vi "Autocross(1Lap).vi"() -> ()   [LabVIEW 2020]
uses:
  Control/AutocrossBestRecordIndicator.ctl
  Control/AutocrossCurrentRecordIndicator(1Lap).ctl
  Control/AutocrossState.ctl
  <vilib>/DAQmx/write.llb/DAQmx Write (Analog DBL 1Chan 1Samp).vi
  <vilib>/DAQmx/read.llb/DAQmx Read (Analog DBL 1Chan 1Samp).vi
  <vilib>/DAQmx/create/channels.llb/DAQmx Create Channel (AO-Voltage-Basic).vi
  <vilib>/DAQmx/create/channels.llb/DAQmx Create Channel (AI-Voltage-Basic).vi
  <vilib>/Utility/file.llb/Read Delimited Spreadsheet (string).vi
  <vilib>/DAQmx/miscellaneous.llb/DAQmx Fill In Error Info.vi
panel:
  out "Event Progress":string[][](table)
  in  "DeviceName":tag
  in  "NextButton":bool
  in  "Ready":bool
  in  "Retry":bool
  out "CurrentRecordIndicator":T1
  out "BestRecordIndicator":T2
  in  "Stop":bool
  # "2017 KSAE Formula Autocross Event"
  # "Time:"
  # "Entry:"
  # "#1"
  # "#2"
  # "#3"
  # "#4"
  # "Univ. :"
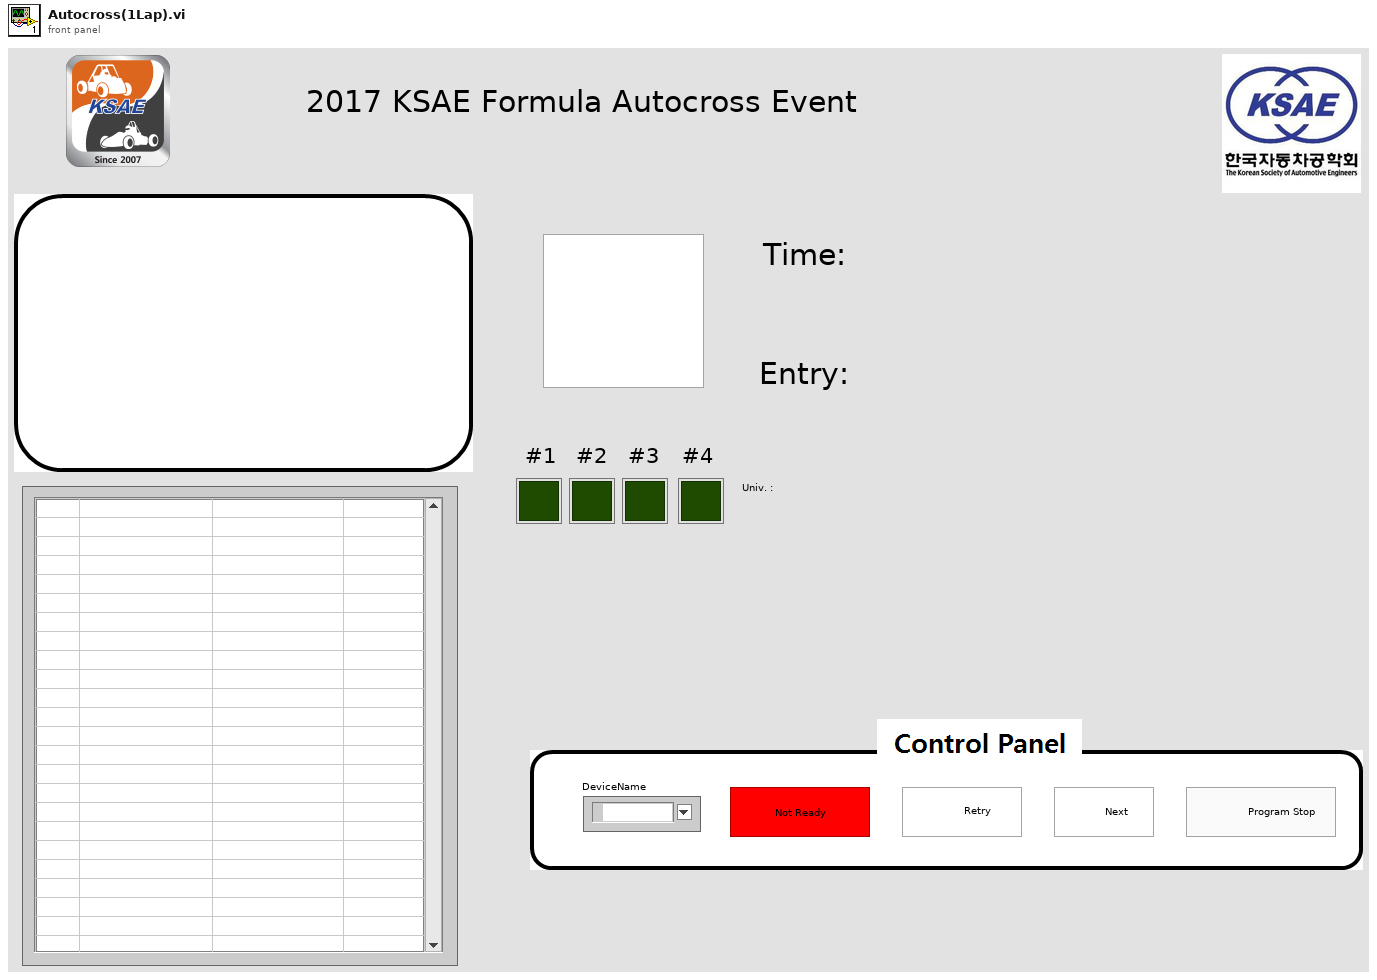
[diagram p1: front panel]
types:
  T1 = typedef "AutocrossCurrentRecordIndicator(1Lap).ctl" = cluster{"Time":string, "CurrentEntry":string, "CurrentUniversity":string, "Flag":picture, "CurrentState":string, "EventCount":cluster{"Attempt-1":bool, "Attempt-2":bool, "Attempt-3":bool, "Attempt-4":bool}}
  T2 = typedef "AutocrossBestRecordIndicator.ctl" = cluster{"BestSchool":string, "BestEntry":string, "BestTime":string}
  T3 = typedef "AutocrossState.ctl" = enum16{"Initial", "InputInfomation", "Ready", "1lap", "2lap", "FinshRunning", "LogRecord", "RenewBestRecord", "ProgramStop"}
  T4 = cluster{"CurrentRecordIndicator":T1, "BestRecordIndicator":T2, "FlageData":cluster{"GreenFlag":picture, "BlueFlag":picture, "RedFlag":picture}, "1LapRefTime":i64, "1LapTime":i64, "State":T3, "EventProgressData":string[][], "EventCount":i32}
  T5 = cluster{"CurrentEntry":string, "CurrentUniversity":string, "CurrentTeam":string}
  T6 = cluster{"Attempt-1":bool, "Attempt-2":bool, "Attempt-3":bool, "Attempt-4":bool}
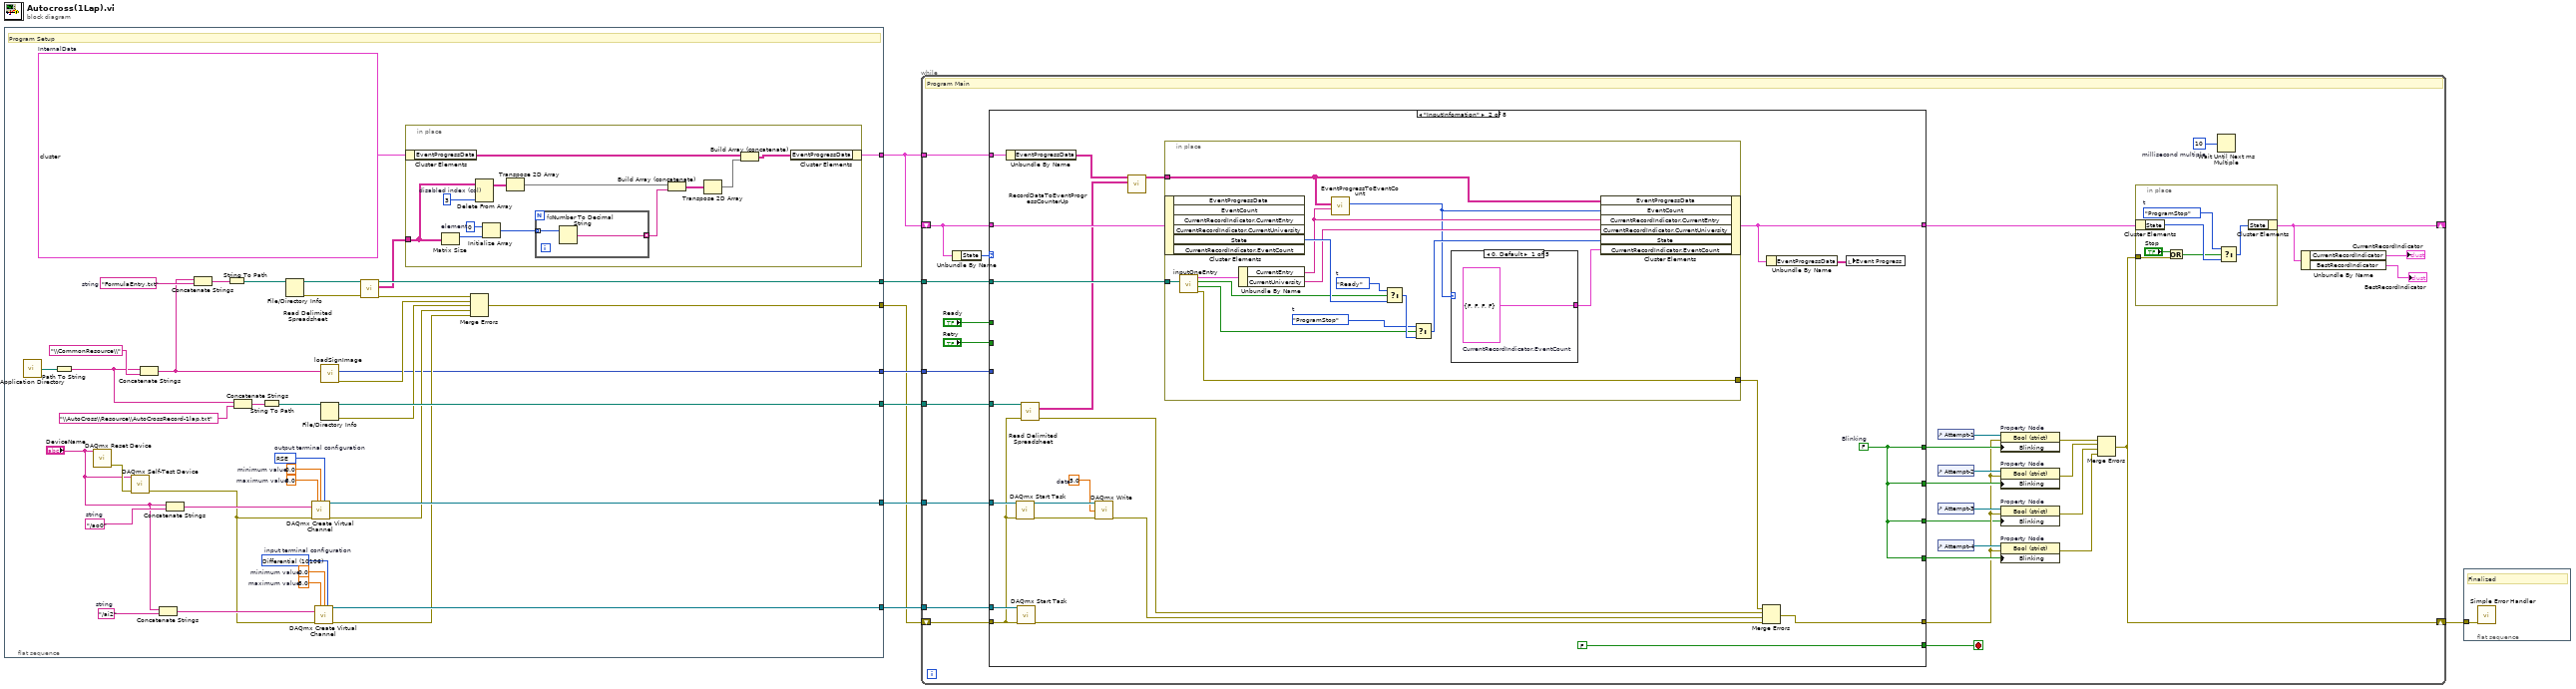
[diagram p0: block diagram]
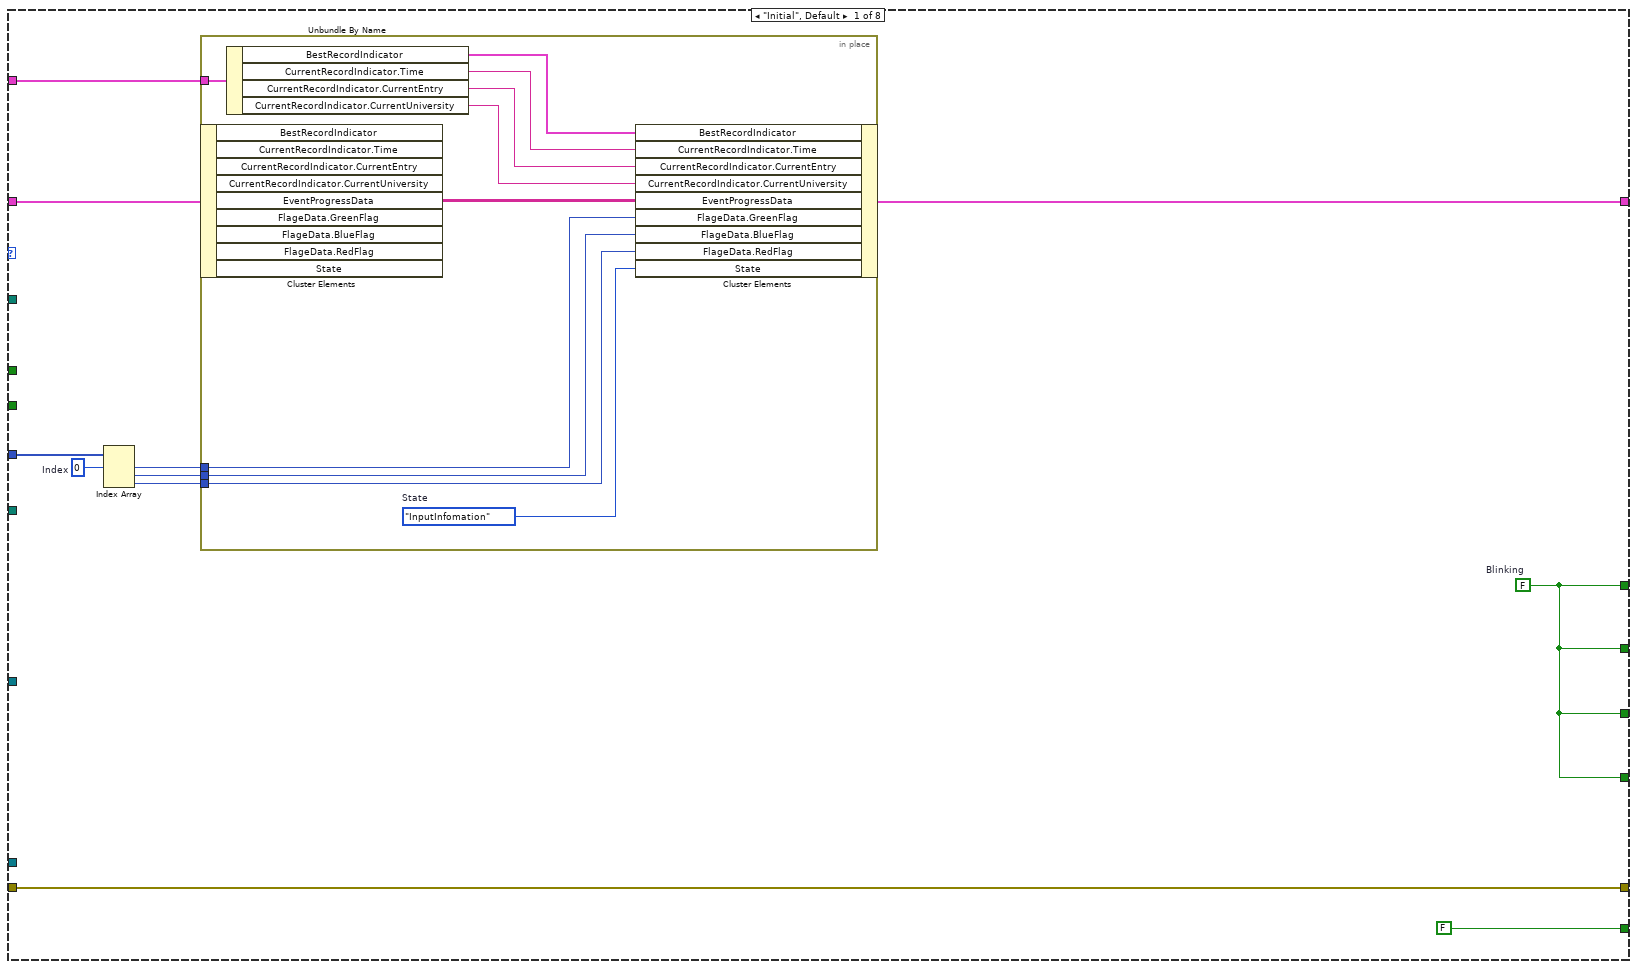
[diagram p2: hidden frame]
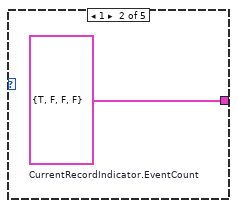
[diagram p3: hidden frame]
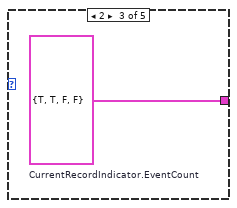
[diagram p4: hidden frame]
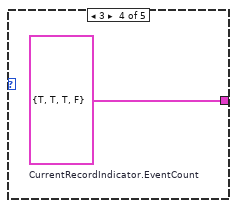
[diagram p5: hidden frame]
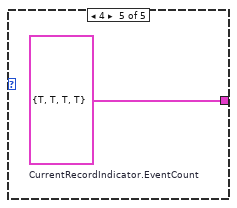
[diagram p6: hidden frame]
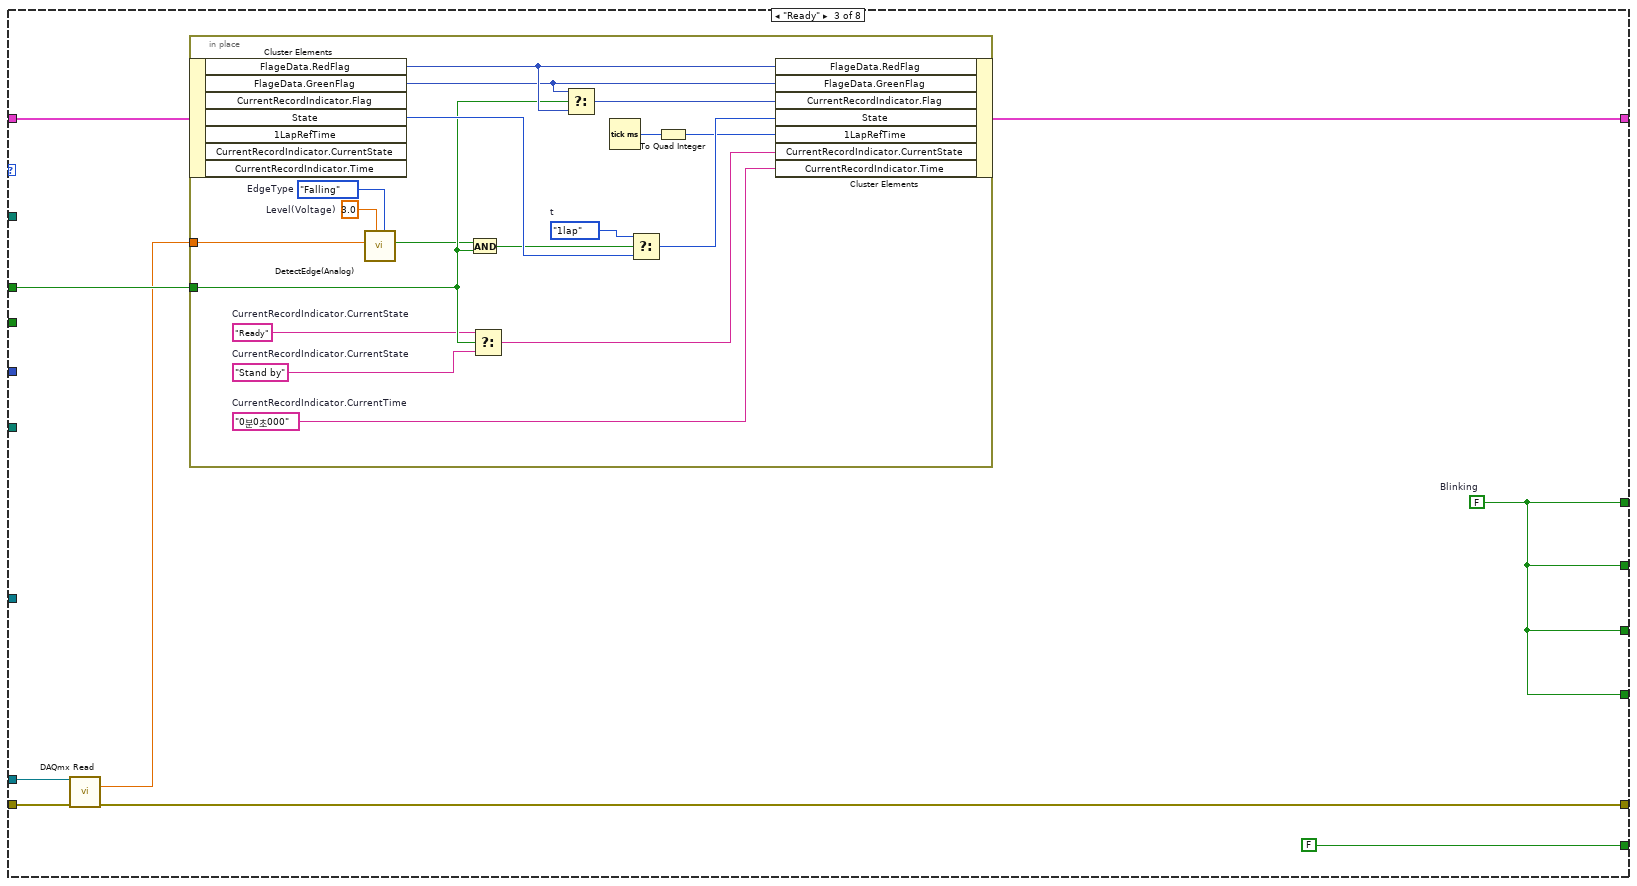
[diagram p7: hidden frame]
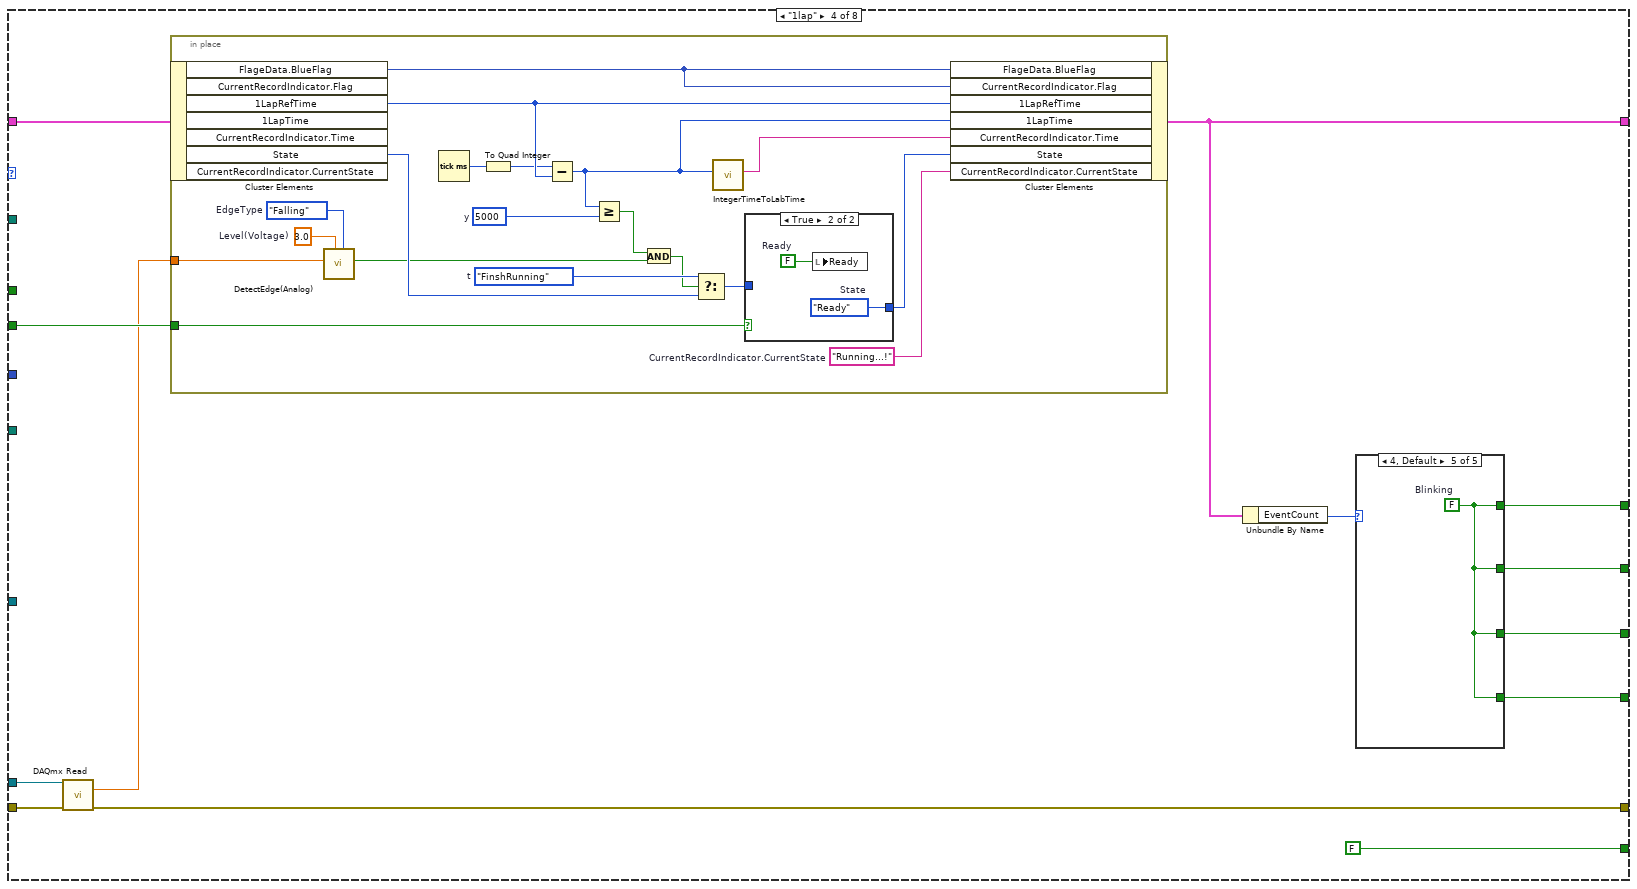
[diagram p8: hidden frame]
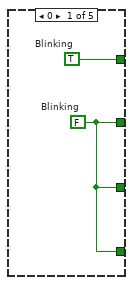
[diagram p9: hidden frame]
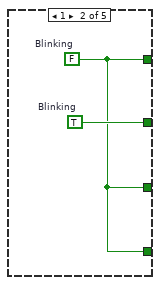
[diagram p10: hidden frame]
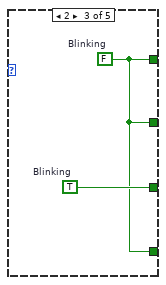
[diagram p11: hidden frame]
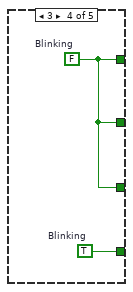
[diagram p12: hidden frame]
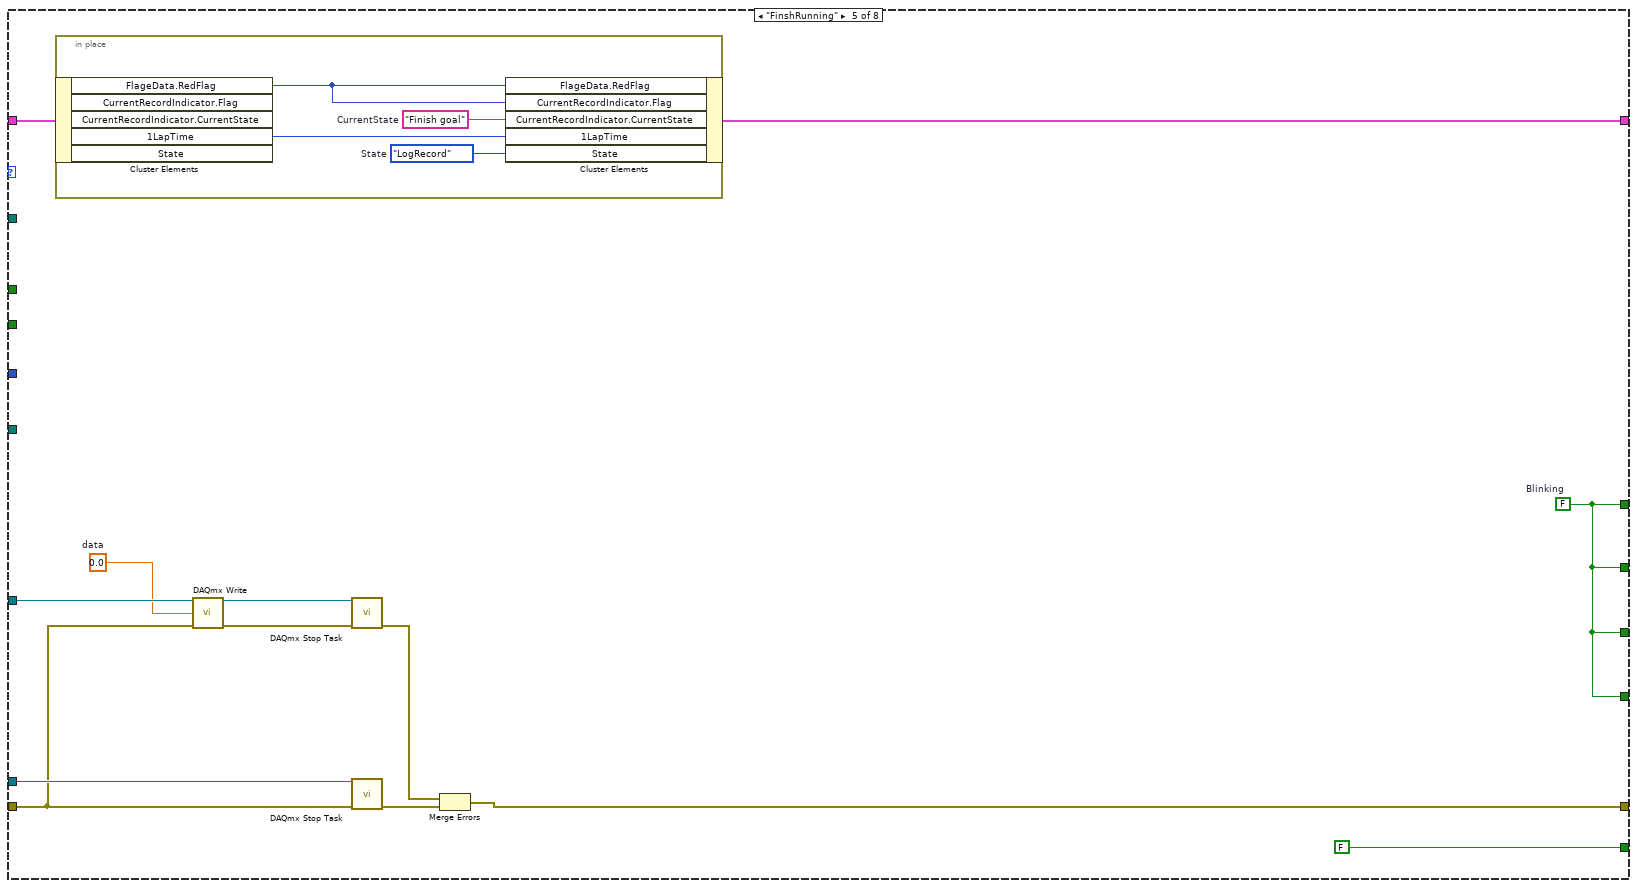
[diagram p14: hidden frame]
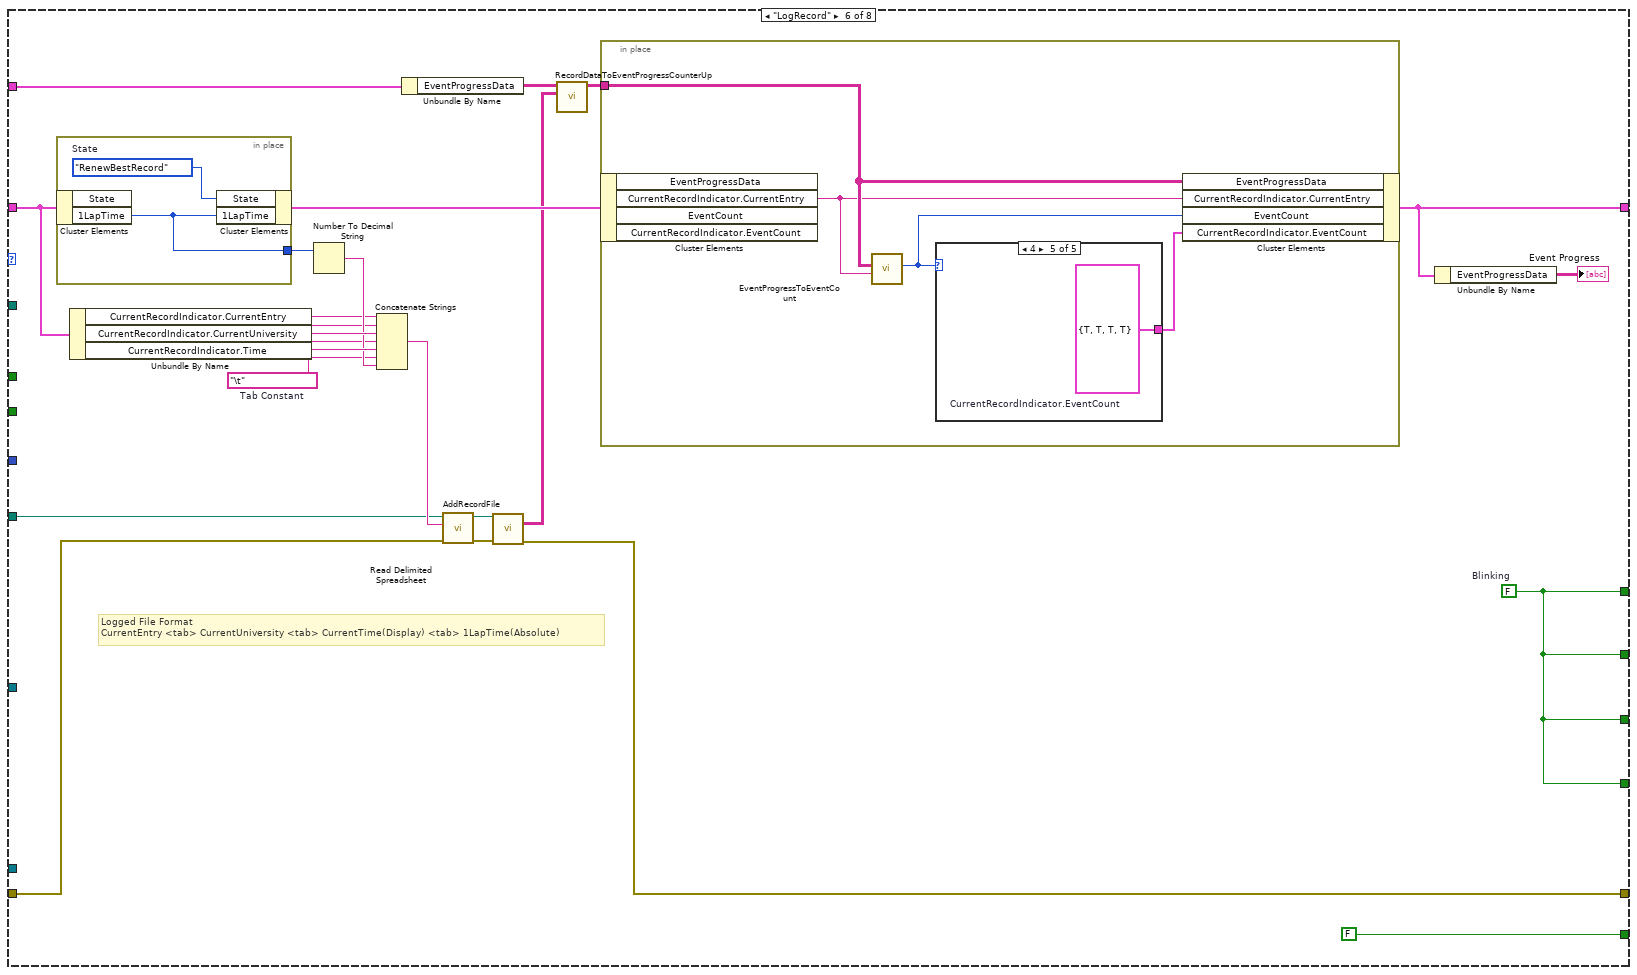
[diagram p15: hidden frame]
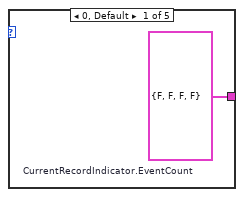
[diagram p16: hidden frame]
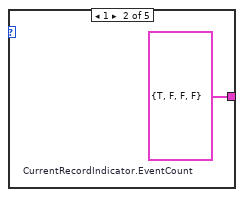
[diagram p17: hidden frame]
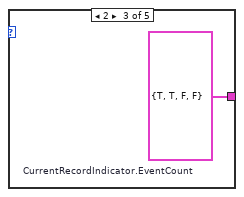
[diagram p18: hidden frame]
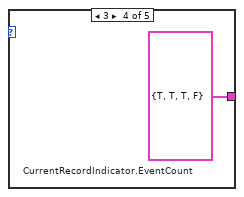
[diagram p19: hidden frame]
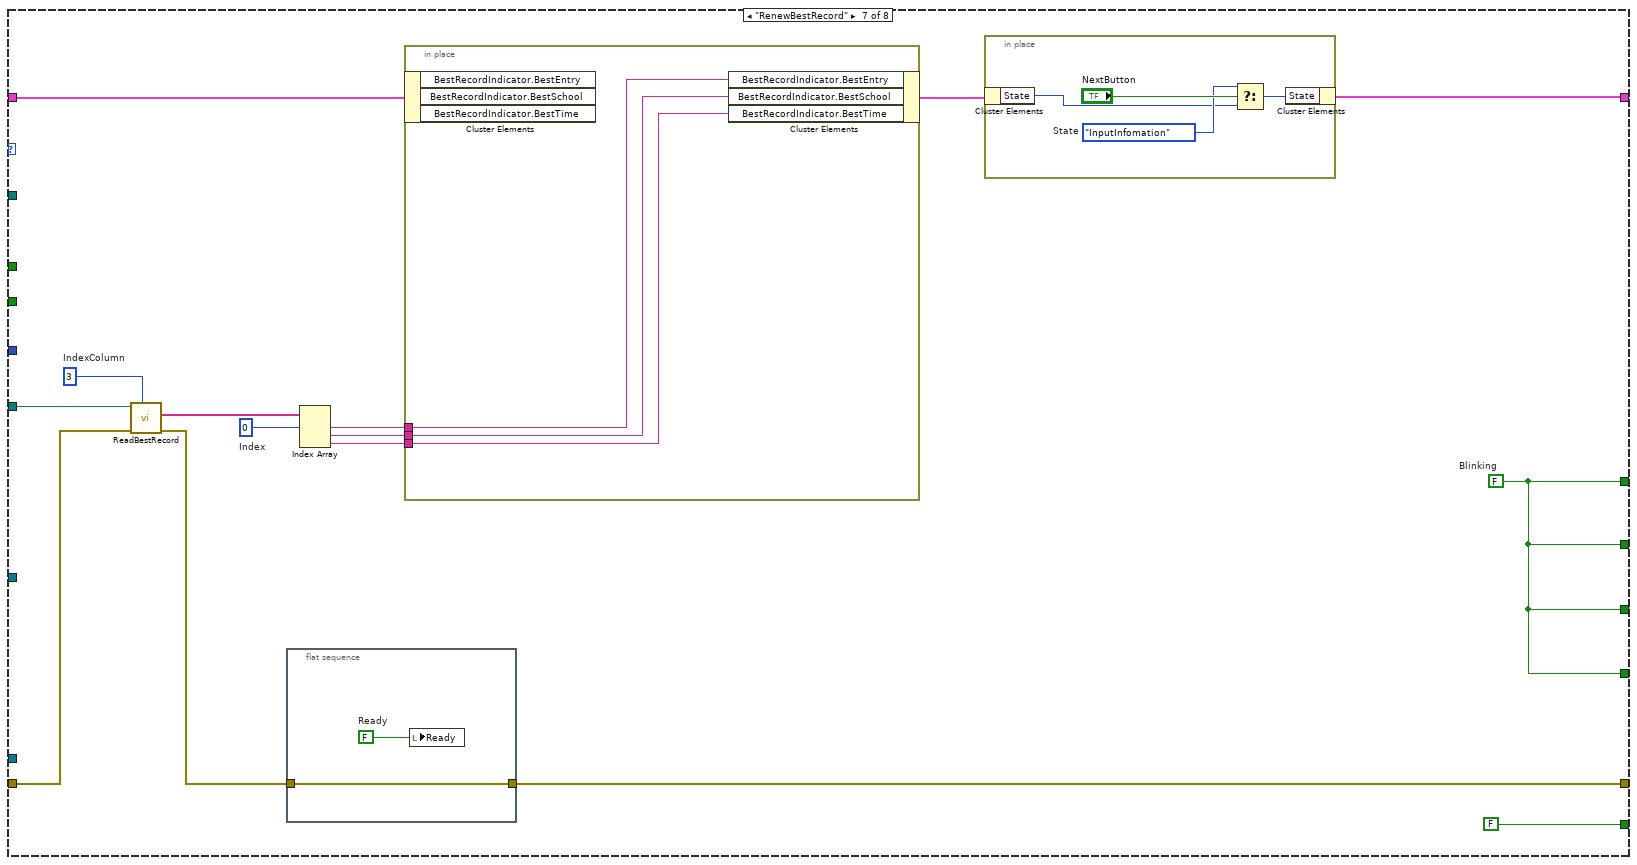
[diagram p20: hidden frame]
diagram:
  n1 = flat-sequence {
    tunnel: [w13] -> w7
    tunnel: [w46] -> w6
    tunnel: [w43] -> w5
    tunnel: [w23] -> w4
    tunnel: [w9] -> w3
    tunnel: [w24] -> w2
    tunnel: [w16] -> w1
    frame #0 {
      w15 = T4 {"CurrentRecordIndicator"={"Time"="", "CurrentEntry"="", "CurrentUniversity"="", "Flag"=bytes[0], "CurrentState"="", "EventCount"={"Attempt-1"=FALSE, "Attempt-2"=FALSE, "Attempt-3"=FALSE, "Attempt-4"=FALSE}}, "BestRecordIndicator"={"BestSchool"="", "BestEntry"="", "BestTime"=""}, "FlageData"={"GreenFlag"=bytes[0], "BlueFlag"=bytes[0], "RedFlag"=bytes[0]}, "1LapRefTime"=0, "1LapTime"=0, "State"=enum."Initial", "EventProgressData"=[["Entry ", "University", "Team", "Event Count"]], "EventCount"=0}  # InternalData
      w31 = "/ai2"  # string
      w32 = "/ao0"  # string
      w33 = "FormulaEntry.txt"  # string
      w40 = 10083 items=["Default"=-1, "RSE"=10083, "Differential"=10106, "Pseudodifferential"=12529]  # output terminal configuration
      w41 = 0.0  # minimum value
      w42 = 5.0  # maximum value
      w45 = 5.0  # maximum value
      w44 = 0.0  # minimum value
      w47 = 10106 items=["default"=-1, "RSE"=10083, "NRSE"=10078, "Differential"=10106, "Pseudodifferential"=12529]  # input terminal configuration
      # "Program Setup"
      n2 = call <vilib>:"Application Directory.vi"() -> ("Application Directory"=w39:path)
      n3 = Path To String(path=w39) -> (string=w35:string)
      n4 = call <vilib>:"DAQmx Reset Device.vi"("device in"="DeviceName") -> ("error out"=w12:errorcluster)  [unwired: 14 in]
      n5 = call <vilib>:"DAQmx Self-Test Device.vi"("device in"="DeviceName", "error in"=w12) -> ("error out"=w11:errorcluster)  [unwired: 13 in]
      n6 = Concatenate Strings "Concatenate Strings"(w35, "\\CommonResource\\") -> (w26:string)
      n7 = Concatenate Strings "Concatenate Strings"("DeviceName", w31) -> (w29:string)
      n8 = Concatenate Strings "Concatenate Strings"("DeviceName", w32) -> (w30:string)
      n9 = Concatenate Strings "Concatenate Strings"(w26, w33) -> (w34:string)
      n10 = String To Path(string=w34) -> (path=w28:path)
      n11 = Concatenate Strings "Concatenate Strings"(w35, "\\AutoCross\\Resource\\AutoCrossRecord-1lap.txt") -> (w37:string)
      n12 = String To Path(string=w37) -> (path=w25:path)
      n13 = File/Directory Info(path=w28) -> (path out=w27:path, error out=w22:errorcluster)  [unwired: 1 in, 5 out]
      n14 = call-poly <vilib>:"DAQmx Create Virtual Channel.vi"("maximum value"=w42, "minimum value"=w41, "output terminal configuration"=w40, "physical channels"=w30, "error in"=w11) -> ("task out"=w43:refnum<k21>, "error out"=w18:errorcluster)  [unwired: 9 in]
      n15 = call-poly <vilib>:"DAQmx Create Virtual Channel.vi"("maximum value"=w45, "minimum value"=w44, "input terminal configuration"=w47, "physical channels"=w29, "error in"=w11) -> ("task out"=w46:refnum<k21>, "error out"=w17:errorcluster)  [unwired: 9 in]
      n16 = File/Directory Info(path=w25) -> (path out=w23:path, error out=w19:errorcluster)  [unwired: 1 in, 5 out]
      n17 = call "loadSignImage.vi"("String"=w26) -> ("outputError"=w20:errorcluster, "SignImageOutput"=w9:picture[])  [unwired: 9 in]
      n18 = call-poly <vilib>:"Read Delimited Spreadsheet.vi"("file path (dialog if empty)"=w27, "error in (no error)"=w22) -> ("new file path (Not A Path if cancelled)"=w24:path, "all rows"=w14:string[][], "error out"=w21:errorcluster)  [unwired: 8 in, 3 out]
      n19 = in-place {
        in-place-border: w14 -> [w56]
        w55 = 3  # disabled index (col)
        w58 = 0  # element
        n20 = in-place-cluster #1(w15) -> ("EventProgressData"=w49:string[][])
        n21 = Matrix Size(0:w56) -> (1:w59:i32)  [unwired: 1 out]
        n22 = Delete From Array "Delete From Array"(array=w56, index (col)=w55) -> (array with subset deleted=w54:string[][])  [unwired: 2 in, 1 out]
        n23 = Initialize Array "Initialize Array"(w58, w59) -> (w57:i32[])
        n24 = Transpose 2D Array(2D array=w54) -> (transposed array=w53:string[][])
        n25 = for {
          tunnel: w57 -> [w61] mode=indexing
          tunnel: [w60] -> w52 mode=indexing
          n26 = Number To Decimal String(number=w61) -> (decimal integer string=w60:string)  [unwired: 1 in]
        }
        n27 = Build Array (concatenate) "Build Array"(w53, w52) -> (w51:string[][])
        n28 = Transpose 2D Array(2D array=w51) -> (transposed array=w50:string[][])
        n29 = Build Array (concatenate) "Build Array"(w49, w50) -> (w48:string[][])
        n30 = in-place-cluster #1("EventProgressData"=w48) -> (w13:T4)
      }
      n31 = Merge Errors "Merge Errors"(w21, w20, w19, w18, w17) -> (w16:errorcluster)
    }
  }
  n32 = while {
    tunnel: w6 -> [w92]
    shift-right: [w85] -> _
    shift-left: w7 -> [w89]
    shift-right: [w63] -> w8
    shift-left: w1 -> [w91]
    tunnel: w7 -> [w83]
    tunnel: w5 -> [w80]
    tunnel: w4 -> [w79]
    tunnel: w3 -> [w77]
    tunnel: w2 -> [w76]
    stop <- w84 stop-if-true
    w78 = u32 10  # millisecond multiple
    # "Program Main"
    n33 = Unbundle By Name(w89) -> ("State"=w90:T3)
    n34 = case shown="\"InputInfomation\"" w90 {
      tunnel: w92 -> [_ w134 w164 w195 w239 _ _ w308]
      tunnel: w91 -> [w94 w115 w163 w194 w228 w255 w289 w302]
      tunnel: w89 -> [w103 w135 w162 w193 w238 w264 w291 w310]
      tunnel: [w102 w117 w161 w188 w237 w245 w281 w309] -> w86
      tunnel: [FALSE FALSE FALSE FALSE FALSE FALSE FALSE TRUE] -> w84
      tunnel: [w94 w132 w160 w192 w232 w248 w279 w304] -> w68
      tunnel: w83 -> [w96 w121 _ _ _ w252 _ _]
      tunnel: "Ready" -> [_ _ w159 _ _ _ _ _]
      tunnel: "Retry" -> [_ _ _ w191 _ _ _ _]
      tunnel: w80 -> [_ w131 _ _ w235 _ _ w305]
      tunnel: w79 -> [_ w123 _ _ _ w258 w278 _]
      tunnel: w77 -> [w95 _ _ _ _ _ _ _]
      tunnel: w76 -> [_ w124 _ _ _ _ _ _]
      tunnel: [w93 w114 w156 w186 w227 w244 w277 w301] -> w71
      tunnel: [w93 w114 w156 w185 w227 w244 w277 w301] -> w70
      tunnel: [w93 w114 w156 w183 w227 w244 w277 w301] -> w69
      tunnel: [w93 w114 w156 w184 w227 w244 w277 w301] -> w62
      frame "Initial", Default {
        w93 = FALSE  # Blinking
        w97 = 0  # Index
        n35 = Index Array "Index Array"(array=w95, index #1=w97) -> (element #1=w100:picture, element #2=w99:picture, element #3=w98:picture)  [unwired: 2 in]
        n36 = in-place {
          in-place-border: w100 -> [w113]
          in-place-border: w99 -> [w112]
          in-place-border: w98 -> [w111]
          in-place-border: w96 -> [w109]
          w110 = AutocrossState."InputInfomation"  # State
          n37 = in-place-cluster #2(w103) -> ("EventProgressData"=w104:string[][])  [unwired: 8 out]
          n38 = Unbundle By Name(w109) -> ("BestRecordIndicator"=w108:T2, "CurrentRecordIndicator.Time"=w107:string, "CurrentRecordIndicator.CurrentEntry"=w105:string, "CurrentRecordIndicator.CurrentUniversity"=w106:string)
          n39 = in-place-cluster #2("BestRecordIndicator"=w108, "CurrentRecordIndicator.Time"=w107, "CurrentRecordIndicator.CurrentEntry"=w105, "CurrentRecordIndicator.CurrentUniversity"=w106, "EventProgressData"=w104, "FlageData.GreenFlag"=w113, "FlageData.BlueFlag"=w112, "FlageData.RedFlag"=w111, "State"=w110) -> (w102:T4)
        }
      }
      frame "InputInfomation" {
        w114 = FALSE  # Blinking
        w126 = 5.0  # data
        n40 = Unbundle By Name(w121) -> ("EventProgressData"=w120:string[][])
        n41 = call <vilib>:"DAQmx Start Task.vi"("task/channels in"=w131, "error in"=w115) -> ("task out"=w129:refnum<k21>, "error out"=w128:errorcluster)  [unwired: 12 in]
        n42 = call <vilib>:"DAQmx Start Task.vi"("task/channels in"=w134, "error in"=w115) -> ("error out"=w133:errorcluster)  [unwired: 12 in, 1 out]
        n43 = call-poly <vilib>:"Read Delimited Spreadsheet.vi"("file path (dialog if empty)"=w123, "error in (no error)"=w115) -> ("all rows"=w119:string[][], "error out"=w122:errorcluster)  [unwired: 8 in, 4 out]
        n44 = call-poly <vilib>:"DAQmx Write.vi"("task/channels in"=w129, "data"=w126, "error in"=w128) -> ("error out"=w127:errorcluster)  [unwired: 10 in, 2 out]
        n45 = call "RecordDataToEventProgressCounterUp.vi"("RecordData"=w119, "EventProgressDataInput"=w120) -> ("EventProgressDataOutput"=w118:string[][])  [unwired: 9 in]
        n46 = in-place {
          in-place-border: [w145] -> w130
          in-place-border: w124 -> [w138]
          in-place-border: w118 -> [w143]
          w147 = AutocrossState."ProgramStop"  # t
          w149 = AutocrossState."Ready"  # t
          n47 = in-place-cluster #3(w135) -> ("State"=w150:T3)  [unwired: 5 out]
          n48 = call "inputOneEntry.vi"("file path (dialog if empty)"=w138) -> ("outputError"=w145:errorcluster, "StopButtonOutput"=w136:bool, "OKButtonOutput"=w137:bool, "CurrentData"=w139:T5)  [unwired: 7 in]
          n49 = Unbundle By Name(w139) -> ("CurrentEntry"=w142:string, "CurrentUniversity"=w144:string)
          n50 = call "EventProgressToEventCount.vi"("CurrentEntry"=w142, "EventProgressDataInput"=w143) -> ("EventCount"=w141:i32)  [unwired: 9 in]
          n51 = Select(t=w149, s=w137, f=w150) -> (s? t:f=w148:T3)
          n52 = Select(t=w147, s=w136, f=w148) -> (s? t:f=w146:T3)
          n53 = case shown="0, Default" w141 {
            tunnel: [w151 w152 w153 w154 w155] -> w140
            frame 0, Default {
              w151 = T6 {"Attempt-1"=FALSE, "Attempt-2"=FALSE, "Attempt-3"=FALSE, "Attempt-4"=FALSE}  # CurrentRecordIndicator.EventCount
            }
            frame 1 {
              w152 = T6 {"Attempt-1"=TRUE, "Attempt-2"=FALSE, "Attempt-3"=FALSE, "Attempt-4"=FALSE}  # CurrentRecordIndicator.EventCount
            }
            frame 2 {
              w153 = T6 {"Attempt-1"=TRUE, "Attempt-2"=TRUE, "Attempt-3"=FALSE, "Attempt-4"=FALSE}  # CurrentRecordIndicator.EventCount
            }
            frame 3 {
              w154 = T6 {"Attempt-1"=TRUE, "Attempt-2"=TRUE, "Attempt-3"=TRUE, "Attempt-4"=FALSE}  # CurrentRecordIndicator.EventCount
            }
            frame 4 {
              w155 = T6 {"Attempt-1"=TRUE, "Attempt-2"=TRUE, "Attempt-3"=TRUE, "Attempt-4"=TRUE}  # CurrentRecordIndicator.EventCount
            }
          }
          n54 = in-place-cluster #3("EventProgressData"=w143, "EventCount"=w141, "CurrentRecordIndicator.CurrentEntry"=w142, "CurrentRecordIndicator.CurrentUniversity"=w144, "State"=w146, "CurrentRecordIndicator.EventCount"=w140) -> (w117:T4)
        }
        n55 = Merge Errors "Merge Errors"(w130, w122, w127, w133) -> (w132:errorcluster)
        n56 = Unbundle By Name(w117) -> ("EventProgressData"=w116:string[][])
        n57 = local write "Event Progress"(w116) -> ()
      }
      frame "Ready" {
        w156 = FALSE  # Blinking
        n58 = call-poly <vilib>:"DAQmx Read.vi"("task/channels in"=w164, "error in"=w163) -> ("data"=w158:dbl, "error out"=w160:errorcluster)  [unwired: 11 in, 1 out]
        n59 = in-place {
          in-place-border: w158 -> [w179]
          in-place-border: w159 -> [w173]
          w165 = enum16{"Rising", "Falling"}."Falling"  # EdgeType
          w170 = "Stand by"  # CurrentRecordIndicator.CurrentState
          w174 = 3.0  # Level(Voltage)
          w167 = "0분0초000"  # CurrentRecordIndicator.CurrentTime
          w171 = "Ready"  # CurrentRecordIndicator.CurrentState
          w180 = AutocrossState."1lap"  # t
          n60 = in-place-cluster #4(w162) -> ("FlageData.RedFlag"=w176:picture, "FlageData.GreenFlag"=w175:picture, "State"=w182:T3)  [unwired: 4 out]
          n61 = call "DetectEdge(Analog).vi"("EdgeType"=w165, "Level(Voltage)"=w174, "Voltage"=w179) -> ("DetectedEdge"=w166:bool)  [unwired: 8 in]
          n62 = And(x=w166, y=w173) -> (x .and. y?=w178:bool)
          n63 = Select(t=w171, s=w173, f=w170) -> (s? t:f=w172:string)
          n64 = Select(t=w175, s=w173, f=w176) -> (s? t:f=w177:picture)
          n65 = Tick Count (ms)() -> (millisecond timer value=w169:u32)
          n66 = Select(t=w180, s=w178, f=w182) -> (s? t:f=w181:T3)
          n67 = To Quad Integer(1:w169) -> (0:w168:i64)
          n68 = in-place-cluster #4("FlageData.RedFlag"=w176, "FlageData.GreenFlag"=w175, "CurrentRecordIndicator.Flag"=w177, "State"=w181, "1LapRefTime"=w168, "CurrentRecordIndicator.CurrentState"=w172, "CurrentRecordIndicator.Time"=w167) -> (w161:T4)
        }
      }
      frame "1lap" {
        n69 = call-poly <vilib>:"DAQmx Read.vi"("task/channels in"=w195, "error in"=w194) -> ("data"=w190:dbl, "error out"=w192:errorcluster)  [unwired: 11 in, 1 out]
        n70 = in-place {
          in-place-border: w191 -> [w209]
          in-place-border: w190 -> [w219]
          w205 = enum16{"Rising", "Falling"}."Falling"  # EdgeType
          w210 = i64 5000  # y
          w218 = 3.0  # Level(Voltage)
          w221 = "Running...!"  # CurrentRecordIndicator.CurrentState
          w223 = AutocrossState."FinshRunning"  # t
          n71 = in-place-cluster #5(w193) -> ("FlageData.BlueFlag"=w222:picture, "1LapRefTime"=w216:i64, "State"=w213:T3)  [unwired: 4 out]
          n72 = call "DetectEdge(Analog).vi"("EdgeType"=w205, "Level(Voltage)"=w218, "Voltage"=w219) -> ("DetectedEdge"=w207:bool)  [unwired: 8 in]
          n73 = Tick Count (ms)() -> (millisecond timer value=w217:u32)
          n74 = To Quad Integer(1:w217) -> (0:w215:i64)
          n75 = Subtract(x=w215, y=w216) -> (x-y=w211:i64)
          n76 = Greater Or Equal?(x=w211, y=w210) -> (x >= y?=w208:bool)
          n77 = And(x=w208, y=w207) -> (x .and. y?=w206:bool)
          n78 = Select(t=w223, s=w206, f=w213) -> (s? t:f=w220:T3)
          n79 = call "IntegerTimeToLabTime.vi"("inputTime(msec)"=w211) -> ("outputTime(mm-ss-sss)"=w214:string)  [unwired: 10 in]
          n80 = case shown="True" w209 {
            tunnel: w220 -> [w224 _]
            tunnel: [w224 w225] -> w212
            frame False {
            }
            frame True {
              w225 = AutocrossState."Ready"  # State
              w226 = FALSE  # Ready
              n81 = local write "Ready"(w226) -> ()
            }
          }
          n82 = in-place-cluster #5("FlageData.BlueFlag"=w222, "CurrentRecordIndicator.Flag"=w222, "1LapRefTime"=w216, "1LapTime"=w211, "CurrentRecordIndicator.Time"=w214, "State"=w212, "CurrentRecordIndicator.CurrentState"=w221) -> (w188:T4)
        }
        n83 = Unbundle By Name(w188) -> ("EventCount"=w187:i32)
        n84 = case shown="4, Default" w187 {
          tunnel: [w197 w198 w200 w202 w204] -> w186
          tunnel: [w196 w199 w200 w202 w204] -> w185
          tunnel: [w196 w198 w201 w202 w204] -> w184
          tunnel: [w196 w198 w200 w203 w204] -> w183
          frame 0 {
            w196 = FALSE  # Blinking
            w197 = TRUE  # Blinking
          }
          frame 1 {
            w199 = TRUE  # Blinking
            w198 = FALSE  # Blinking
          }
          frame 2 {
            w201 = TRUE  # Blinking
            w200 = FALSE  # Blinking
          }
          frame 3 {
            w203 = TRUE  # Blinking
            w202 = FALSE  # Blinking
          }
          frame 4, Default {
            w204 = FALSE  # Blinking
          }
        }
      }
      frame "FinshRunning" {
        w227 = FALSE  # Blinking
        w230 = 0.0  # data
        n85 = in-place {
          w241 = AutocrossState."LogRecord"  # State
          w242 = "Finish goal"  # CurrentState
          n86 = in-place-cluster #6(w238) -> ("FlageData.RedFlag"=w243:picture, "1LapTime"=w240:i64)  [unwired: 3 out]
          n87 = in-place-cluster #6("FlageData.RedFlag"=w243, "CurrentRecordIndicator.Flag"=w243, "CurrentRecordIndicator.CurrentState"=w242, "1LapTime"=w240, "State"=w241) -> (w237:T4)
        }
        n88 = call-poly <vilib>:"DAQmx Write.vi"("task/channels in"=w235, "data"=w230, "error in"=w228) -> ("task out"=w234:refnum<k21>, "error out"=w233:errorcluster)  [unwired: 10 in, 1 out]
        n89 = call <vilib>:"DAQmx Stop Task.vi"("task/channels in"=w234, "error in"=w233) -> ("error out"=w231:errorcluster)  [unwired: 12 in, 1 out]
        n90 = call <vilib>:"DAQmx Stop Task.vi"("task/channels in"=w239, "error in"=w228) -> ("error out"=w236:errorcluster)  [unwired: 12 in, 1 out]
        n91 = Merge Errors "Merge Errors"(w231, w236) -> (w232:errorcluster)
      }
      frame "LogRecord" {
        w244 = FALSE  # Blinking
        w259 = "\t"  # Tab Constant
        # "Logged File Format\nCurrentEntry <tab> CurrentUniversity <tab> CurrentTime(Display) <tab> 1LapTime(Absolute)"
        n92 = in-place {
          in-place-border: [w275] -> w254
          w276 = AutocrossState."RenewBestRecord"  # State
          n93 = in-place-cluster #7(w264) -> ("1LapTime"=w275:i64)  [unwired: 1 out]
          n94 = in-place-cluster #7("State"=w276, "1LapTime"=w275) -> (w253:T4)
        }
        n95 = Unbundle By Name(w264) -> ("CurrentRecordIndicator.CurrentEntry"=w257:string, "CurrentRecordIndicator.CurrentUniversity"=w263:string, "CurrentRecordIndicator.Time"=w262:string)
        n96 = Number To Decimal String(number=w254) -> (decimal integer string=w260:string)  [unwired: 1 in]
        n97 = Concatenate Strings "Concatenate Strings"(w257, w259, w263, w259, w262, w259, w260) -> (w261:string)
        n98 = Unbundle By Name(w252) -> ("EventProgressData"=w251:string[][])
        n99 = call "AddRecordFile.vi"("에러 입력"=w255, "LabTime"=w261, "파일 경로(대화 상자 사용)"=w258) -> ("에러 출력"=w249:errorcluster, "경로"=w250:path)  [unwired: 7 in]
        n100 = call-poly <vilib>:"Read Delimited Spreadsheet.vi"("file path (dialog if empty)"=w250, "error in (no error)"=w249) -> ("all rows"=w247:string[][], "error out"=w248:errorcluster)  [unwired: 8 in, 4 out]
        n101 = call "RecordDataToEventProgressCounterUp.vi"("RecordData"=w247, "EventProgressDataInput"=w251) -> ("EventProgressDataOutput"=w246:string[][])  [unwired: 9 in]
        n102 = in-place {
          in-place-border: w246 -> [w269]
          n103 = in-place-cluster #8(w253) -> ("CurrentRecordIndicator.CurrentEntry"=w268:string)  [unwired: 3 out]
          n104 = call "EventProgressToEventCount.vi"("CurrentEntry"=w268, "EventProgressDataInput"=w269) -> ("EventCount"=w267:i32)  [unwired: 9 in]
          n105 = case shown="4" w267 {
            tunnel: [w270 w271 w272 w273 w274] -> w266
            frame 0, Default {
              w270 = T6 {"Attempt-1"=FALSE, "Attempt-2"=FALSE, "Attempt-3"=FALSE, "Attempt-4"=FALSE}  # CurrentRecordIndicator.EventCount
            }
            frame 1 {
              w271 = T6 {"Attempt-1"=TRUE, "Attempt-2"=FALSE, "Attempt-3"=FALSE, "Attempt-4"=FALSE}  # CurrentRecordIndicator.EventCount
            }
            frame 2 {
              w272 = T6 {"Attempt-1"=TRUE, "Attempt-2"=TRUE, "Attempt-3"=FALSE, "Attempt-4"=FALSE}  # CurrentRecordIndicator.EventCount
            }
            frame 3 {
              w273 = T6 {"Attempt-1"=TRUE, "Attempt-2"=TRUE, "Attempt-3"=TRUE, "Attempt-4"=FALSE}  # CurrentRecordIndicator.EventCount
            }
            frame 4 {
              w274 = T6 {"Attempt-1"=TRUE, "Attempt-2"=TRUE, "Attempt-3"=TRUE, "Attempt-4"=TRUE}  # CurrentRecordIndicator.EventCount
            }
          }
          n106 = in-place-cluster #8("EventProgressData"=w269, "CurrentRecordIndicator.CurrentEntry"=w268, "EventCount"=w267, "CurrentRecordIndicator.EventCount"=w266) -> (w245:T4)
        }
        n107 = Unbundle By Name(w245) -> ("EventProgressData"=→"Event Progress":string[][])
      }
      frame "RenewBestRecord" {
        w277 = FALSE  # Blinking
        w283 = 3  # IndexColumn
        w284 = 0  # Index
        n108 = call "ReadBestRecord.vi"("IndexColumn"=w283, "ErrorInput"=w289, "FilepathInput"=w278) -> ("ErrorOutput"=w280:errorcluster, "Data"=w288:string[])  [unwired: 6 in, 1 out]
        n109 = flat-sequence {
          tunnel: w280 -> [w292]
          tunnel: [w292] -> w279
          frame #0 {
            w293 = FALSE  # Ready
            n110 = local write "Ready"(w293) -> ()
          }
        }
        n111 = Index Array "Index Array"(array=w288, index #1=w284) -> (element #1=w287:string, element #2=w286:string, element #3=w285:string)  [unwired: 2 in]
        n112 = in-place {
          in-place-border: w287 -> [w300]
          in-place-border: w286 -> [w299]
          in-place-border: w285 -> [w298]
          n113 = in-place-cluster #9(w291) -> ()  [unwired: 3 out]
          n114 = in-place-cluster #9("BestRecordIndicator.BestEntry"=w300, "BestRecordIndicator.BestSchool"=w299, "BestRecordIndicator.BestTime"=w298) -> (w282:T4)
        }
        n115 = in-place {
          w296 = AutocrossState."InputInfomation"  # State
          n116 = in-place-cluster #10(w282) -> ("State"=w294:T3)
          n117 = Select(t=w296, s="NextButton", f=w294) -> (s? t:f=w295:T3)
          n118 = in-place-cluster #10("State"=w295) -> (w281:T4)
        }
      }
      frame "ProgramStop" {
        w301 = FALSE  # Blinking
        n119 = call <vilib>:"DAQmx Clear Task.vi"("task in"=w305, "error in"=w302) -> ("error out"=w303:errorcluster)  [unwired: 13 in]
        n120 = call <vilib>:"DAQmx Clear Task.vi"("task in"=w308, "error in"=w302) -> ("error out"=w307:errorcluster)  [unwired: 13 in]
        n121 = in-place {
          w315 = "Halted Program"  # CurrentRecordIndicator.CurrentState
          n122 = in-place-cluster #11(w310) -> ("FlageData.RedFlag"=w314:picture)  [unwired: 2 out]
          n123 = in-place-cluster #11("FlageData.RedFlag"=w314, "CurrentRecordIndicator.Flag"=w314, "CurrentRecordIndicator.CurrentState"=w315) -> (w309:T4)
        }
        n124 = flat-sequence {
          tunnel: w307 -> [w313]
          tunnel: [w313] -> w306
          frame #0 {
            w312 = FALSE  # Ready
            n125 = local write "Ready"(w312) -> ()
          }
        }
        n126 = Merge Errors "Merge Errors"(w303, w306) -> (w304:errorcluster)
      }
    }
    n127 = control-ref of="Attempt-1"() -> (w75:refnum<vi>)
    n128 = control-ref of="Attempt-2"() -> (w74:refnum<vi>)
    n129 = control-ref of="Attempt-3"() -> (w73:refnum<vi>)
    n130 = control-ref of="Attempt-4"() -> (w72:refnum<vi>)
    n131 = property on="Property Node" class="Bool (strict)"(reference=w75, error in=w68, "Blinking"=w71) -> (error out=w67:errorcluster)  [unwired: 1 out]
    n132 = property on="Property Node" class="Bool (strict)"(reference=w74, error in=w68, "Blinking"=w70) -> (error out=w66:errorcluster)  [unwired: 1 out]
    n133 = property on="Property Node" class="Bool (strict)"(reference=w73, error in=w68, "Blinking"=w62) -> (error out=w65:errorcluster)  [unwired: 1 out]
    n134 = property on="Property Node" class="Bool (strict)"(reference=w72, error in=w68, "Blinking"=w69) -> (error out=w64:errorcluster)  [unwired: 1 out]
    n135 = Merge Errors "Merge Errors"(w67, w66, w65, w64) -> (w63:errorcluster)
    n136 = in-place {
      in-place-border: w63 -> [w316]
      w318 = AutocrossState."ProgramStop"  # t
      n137 = in-place-cluster #12(w86) -> ("State"=w320:T3)
      n138 = Or(x="Stop", y=w316) -> (x .or. y?=w317:bool)
      n139 = Select(t=w318, s=w317, f=w320) -> (s? t:f=w319:T3)
      n140 = in-place-cluster #12("State"=w319) -> (w85:T4)
    }
    n141 = Wait Until Next ms Multiple(millisecond multiple=w78) -> ()  [unwired: 1 out]
    n142 = Unbundle By Name(w85) -> ("CurrentRecordIndicator"=→"CurrentRecordIndicator":T1, "BestRecordIndicator"=→"BestRecordIndicator":T2)
  }
  n143 = flat-sequence {
    tunnel: w8 -> [w322]
    frame #0 {
      # "Finalized"
      n144 = call <vilib>:"Simple Error Handler.vi"("error in (no error)"=w322) -> ()  [unwired: 4 in, 5 out]
    }
  }
